vi "ID_empty.vi"(7 "ID (Profile)":string="Profile", 10 "ID in":string, 11 "Profile NO":u8) -> (2 "ID out":string, 3 "Profile NO out":string)   [LabVIEW 2019, in "STAV lib.lvlib"]
uses:
  STAV lib.lvlib
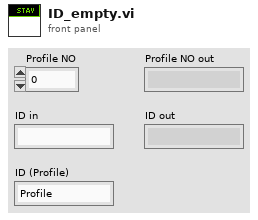
[diagram p1: front panel]
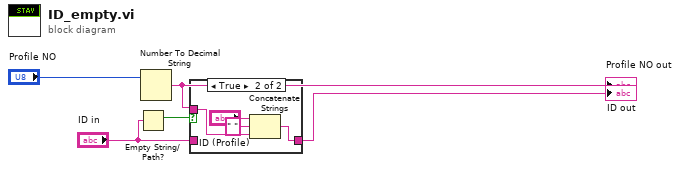
[diagram p0: block diagram]
diagram:
  n1 = Empty String/Path?(string/path="ID in") -> (empty?=w2:bool)
  n2 = Number To Decimal String(number="Profile NO") -> (decimal integer string=w3:string)  [unwired: 1 in]
  "Profile NO out" <- w3
  n3 = case shown="True" w2 {
    tunnel: w3 -> [_ w10]
    tunnel: "ID in" -> [w6 _]
    tunnel: [w6 w9] -> w5
    frame False {
    }
    frame True {
      n4 = Concatenate Strings("ID (Profile)", " " ("string"), w10) -> (w9:string)
    }
  }
  "ID out" <- w5
